vi "Rhythm-Create Envelope.vi"(0 "Data in":T1, 9 "Npts":i32, 11 "error in (no error)":errorcluster) -> (4 "Data out":T1, 8 "Y":dbl[](array[numeric]), 15 "error out":errorcluster)   [LabVIEW 2020]
uses:
  Rhythm-Data.ctl
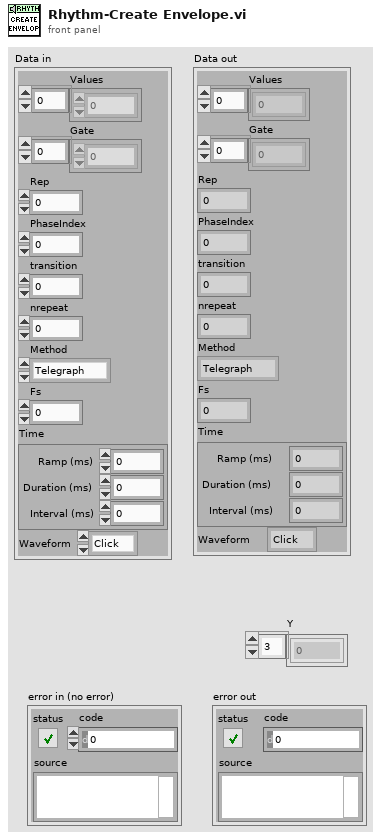
[diagram p1: front panel]
types:
  T1 = typedef "Rhythm-Data.ctl" = cluster{"Values":dbl[], "Gate":dbl[], "Rep":i32, "PhaseIndex":i32, "transition":i32, "nrepeat":i32, "Method":enum16{"Telegraph", "Interval"}, "Fs":dbl, "Time":cluster{"Ramp (ms)":dbl, "Duration (ms)":dbl, "Interval (ms)":dbl}, "Waveform":enum16{"Click", "Noise"}}
  T2 = cluster{"Ramp (ms)":dbl, "Duration (ms)":dbl, "Interval (ms)":dbl}
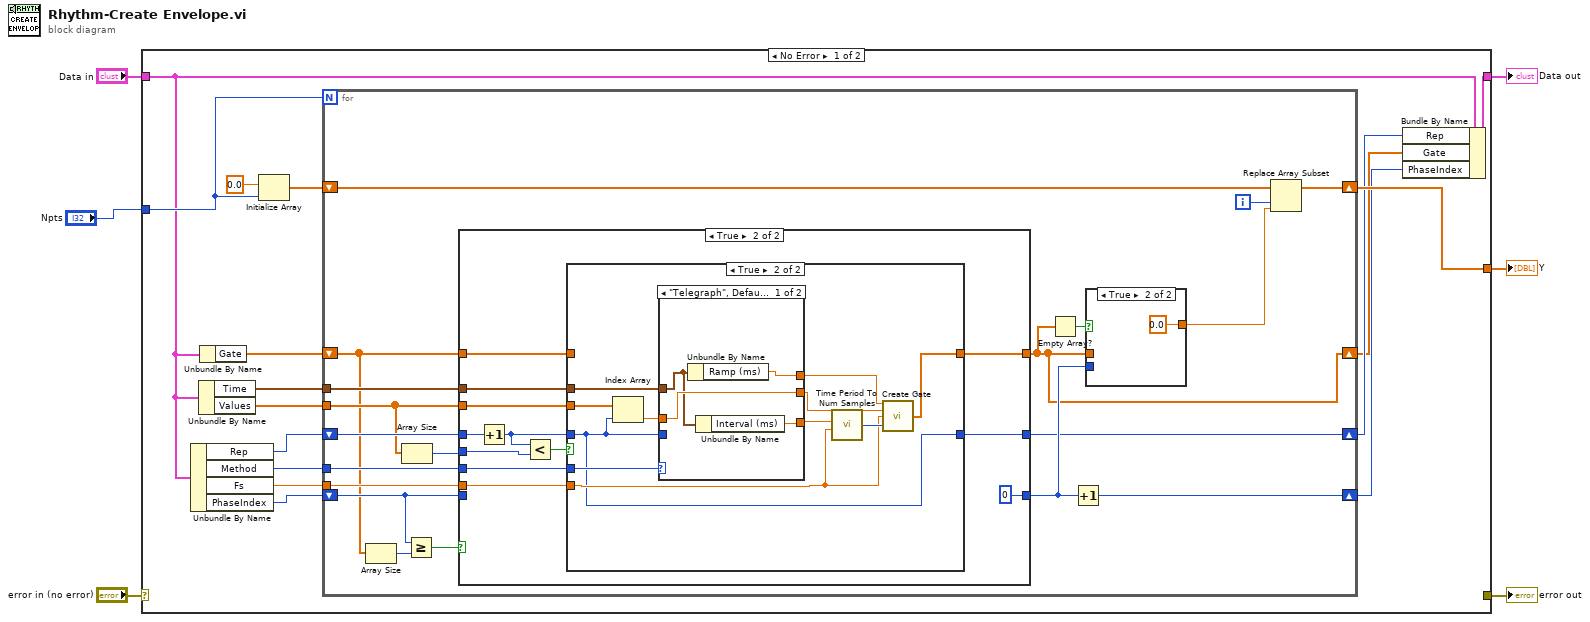
[diagram p0: block diagram]
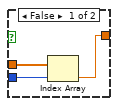
[diagram p2: hidden frame]
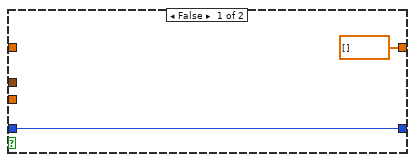
[diagram p4: hidden frame]
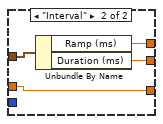
[diagram p5: hidden frame]
diagram:
  n1 = case shown="No Error" "error in (no error)" {
    selector: "error in (no error)" -> [_ w83]
    tunnel: "Data in" -> [w11 w82]
    tunnel: [w18 w82] -> w4
    tunnel: [_ w83] -> w5
    tunnel: "Npts" -> [w16 _]
    tunnel: [w20 _] -> w1
    frame No Error {
      n2 = Unbundle By Name(w11) -> ("Rep"=w14:i32, "Method"=w15:enum16{"Telegraph", "Interval"}, "Fs"=w13:dbl, "PhaseIndex"=w19:i32)
      n3 = Unbundle By Name(w11) -> ("Time"=w12:T2, "Values"=w17:dbl[])
      n4 = Unbundle By Name(w11) -> ("Gate"=w10:dbl[])
      n5 = Initialize Array(0.0, w16) -> (w21:dbl[])
      n6 = for {
        N: w16 -> [_]
        shift-right: [w29] -> w20
        shift-left: w21 -> [w35]
        tunnel: w17 -> [w26]
        tunnel: w15 -> [w39]
        shift-right: [w28] -> w9
        shift-left: w14 -> [w38]
        tunnel: w13 -> [w37]
        tunnel: w12 -> [w36]
        shift-right: [w27] -> w8
        shift-left: w10 -> [w23]
        shift-right: [w30] -> w7
        shift-left: w19 -> [w40]
        i -> [w34]
        n7 = Array Size(array=w23) -> (size(s)=w24:i32)
        n8 = Array Size(array=w26) -> (size(s)=w25:i32)
        n9 = Greater Or Equal?(x=w40, y=w24) -> (x >= y?=w41:bool)
        n10 = case shown="True" w41 {
          tunnel: [w48 0] -> w31
          tunnel: w40 -> [w48 _]
          tunnel: w39 -> [_ w56]
          tunnel: w38 -> [w46 w59]
          tunnel: w25 -> [_ w58]
          tunnel: w26 -> [_ w54]
          tunnel: w37 -> [_ w53]
          tunnel: w36 -> [_ w52]
          tunnel: w23 -> [w47 w51]
          tunnel: [w47 w50] -> w27
          tunnel: [w46 w49] -> w28
          frame False {
          }
          frame True {
            n11 = Increment(x=w59) -> (x+1=w55:i32)
            n12 = Less?(x=w55, y=w58) -> (x < y?=w57:bool)
            n13 = case shown="True" w57 {
              tunnel: w56 -> [_ w73]
              tunnel: w55 -> [w61 w63]
              tunnel: w54 -> [_ w72]
              tunnel: w53 -> [_ w64]
              tunnel: w52 -> [_ w70]
              tunnel: w51 -> [_ _]
              tunnel: [dbl[] [] ("Gate") w65] -> w50
              tunnel: [w61 w63] -> w49
              frame False {
              }
              frame True {
                n14 = Index Array(array=w72, index=w63) -> (element=w71:dbl)
                n15 = case shown="\"Telegraph\", Default" w73 {
                  tunnel: w63 -> [_ _]
                  tunnel: w71 -> [w77 w78]
                  tunnel: [w74 w78] -> w67
                  tunnel: w70 -> [w75 w81]
                  tunnel: [w76 w80] -> w69
                  tunnel: [w77 w79] -> w68
                  frame "Telegraph", Default {
                    n16 = Unbundle By Name(w75) -> ("Ramp (ms)"=w76:dbl)
                    n17 = Unbundle By Name(w75) -> ("Interval (ms)"=w74:dbl)
                  }
                  frame "Interval" {
                    n18 = Unbundle By Name(w81) -> ("Ramp (ms)"=w80:dbl, "Duration (ms)"=w79:dbl)
                  }
                }
                n19 = call "Time Period To Num Samples.vi"("Duration (ms)"=w67, "Sampling rate (Hz)"=w64) -> ("Samples"=w66:i32)  [unwired: 5 in]
                n20 = call "Create Gate.vi"("Ramp (ms)"=w69, "Duration (ms)"=w68, "Sampling Rate (Hz)"=w64, "Npts"=w66) -> ("Gate"=w65:dbl[])  [unwired: 10 in, 1 out]
              }
            }
          }
        }
        n21 = Empty Array?(array=w27) -> (empty?=w33:bool)
        n22 = Increment(x=w31) -> (x+1=w30:i32)
        n23 = case shown="True" w33 {
          tunnel: [w42 0.0] -> w32
          tunnel: w27 -> [w44 _]
          tunnel: w31 -> [w43 _]
          frame False {
            n24 = Index Array(array=w44, index=w43) -> (element=w42:dbl)
          }
          frame True {
          }
        }
        n25 = Replace Array Subset(array=w35, new element=w32, index=w34) -> (w29:dbl[])
      }
      n26 = Bundle By Name(cluster=w11, "Rep"=w9, "Gate"=w8, "PhaseIndex"=w7) -> (w18:T1)
    }
    frame Error {
    }
  }
  "error out" <- w5
  "Data out" <- w4
  "Y" <- w1
